vi "CAL_FLOW_SENSOR 2016.vi"(7 "Array in":refnum<k24>[](array[refnum]), 8 "error in (no error)":errorcluster, 9 "Descriptions":string[](array[string]), 11 "flow_slope_IN":dbl=51.35 format="%.2f") -> (0 "error out":errorcluster, 2 "Sensor Cluster":T1, 3 "flow_slope\nmL/min":dbl=51.35 format="%.2f", 5 "Array out":refnum<k24>[](array[refnum]))   [LabVIEW 2016]
uses:
  C:/Program Files (x86)/National Instruments/LabVIEW 2016/vi.lib/ULx/ULx_LV.dll
  Waterloo DAQ/controls/MCC DAQ Readings.ctl
  KPRO_lv2015/ad interface/Global_SIM_switch.vi
  KPRO_lv2015/Kpro Globals.vi
panel:
  out "Flow":dbl format="%.2f"
  in  "stop":bool
  in  "start":bool
  # "FLOW SENSOR CALIBRATION"
  # "Start Kpro flow. Allow the flow to equilibrate."
  # "After flow has equilibrated,  Press Start, simultaneously move Kpro effluent into graduated cylinder."
  # "Press Stop when 100 mL of water has been collected."
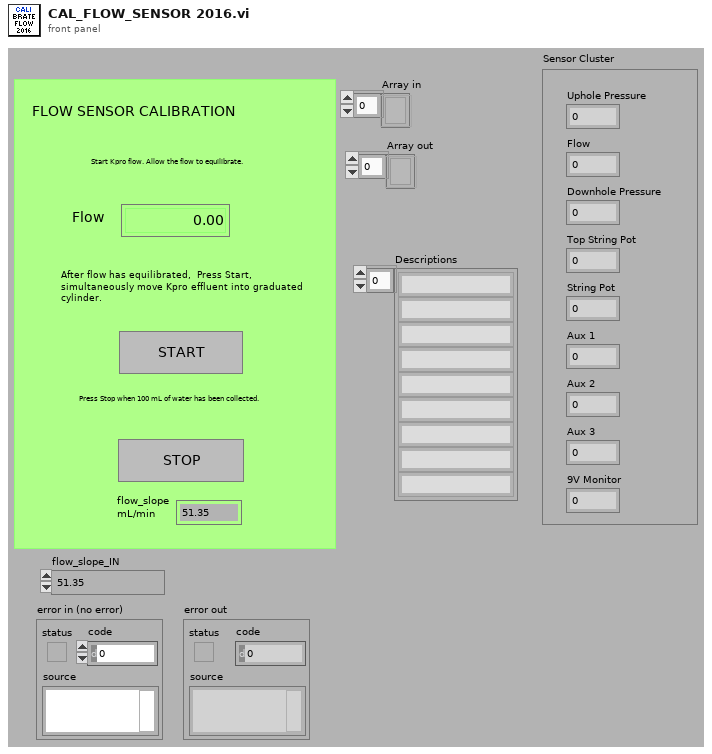
[diagram p1: front panel]
types:
  T1 = typedef "MCC DAQ Readings.ctl" = cluster{"Uphole Pressure":dbl, "Flow":dbl, "Downhole Pressure":dbl, "Top String Pot":dbl, "String Pot":dbl, "Aux 1":dbl, "Aux 2":dbl, "Aux 3":dbl, "9V Monitor":dbl}
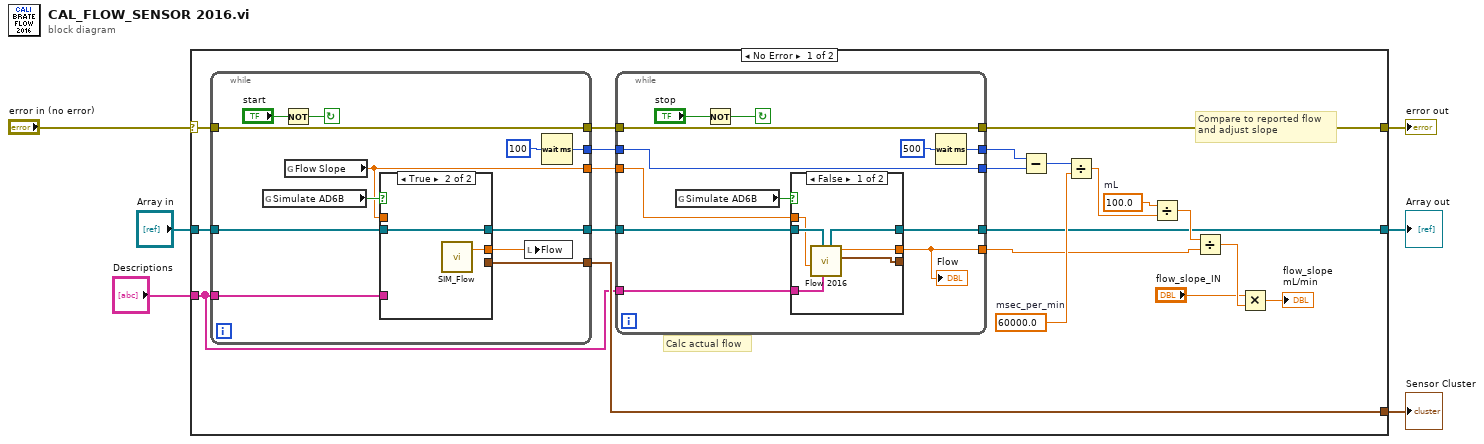
[diagram p0: block diagram]
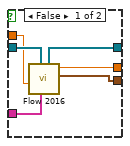
[diagram p2: hidden frame]
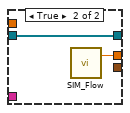
[diagram p3: hidden frame]
diagram:
  n1 = case shown="No Error" "error in (no error)" {
    selector: "error in (no error)" -> [w27 w69]
    tunnel: [w25 w69] -> w6
    tunnel: "Descriptions" -> [w10 _]
    tunnel: "Array in" -> [w12 w68]
    tunnel: [w11 _] -> w2
    tunnel: [w8 w68] -> w1
    frame No Error {
      w20 = 60000.0  # msec_per_min
      w21 = 100.0  # mL
      # "Compare to reported flow\nand adjust slope"
      # "Calc actual flow"
      n2 = while {
        tunnel: [w35] -> w26
        tunnel: w27 -> [w35]
        tunnel: [w36] -> w24
        tunnel: w10 -> [w32]
        tunnel: w12 -> [w31]
        tunnel: [w30] -> w11
        tunnel: [w29] -> w9
        tunnel: [w28] -> w7
        stop <- w38 continue-if-true
        n3 = global read "Global_SIM_switch.vi" "Simulate AD6B"() -> (w34:bool)
        n4 = Not(x="start") -> (.not. x?=w38:bool)
        n5 = global read "Kpro Globals.vi" "Flow Slope"() -> (w28:dbl)
        n6 = case shown="True" w34 {
          tunnel: [w42 w47] -> w33
          tunnel: w32 -> [w45 _]
          tunnel: w31 -> [w44 w46]
          tunnel: [w43 _] -> w30
          tunnel: w28 -> [w41 _]
          tunnel: [w40 w46] -> w29
          frame False {
            n7 = call "Flow 2016.vi"("Descriptions"=w45, "Array in"=w44, "Flow Slope"=w41) -> ("Sensor Cluster"=w43:T1, "Flow (ml/min)"=w42:dbl, "Array out"=w40:refnum<k24>[])  [unwired: 5 in]
          }
          frame True {
            n8 = call "SIM_Flow.vi"() -> ("Flow (ml/min)"=w47:dbl)  [unwired: 3 in]
          }
        }
        n9 = local write "Flow"(w33) -> ()
        n10 = Wait (ms)(milliseconds to wait=u32 100) -> (millisecond timer value=w36:u32)
      }
      n11 = while {
        tunnel: [w49] -> w13
        tunnel: w24 -> [w54]
        tunnel: [w54] -> w22
        tunnel: w26 -> [w55]
        tunnel: [w55] -> w25
        tunnel: [w57] -> w23
        tunnel: w10 -> [w52]
        tunnel: w9 -> [w51]
        tunnel: [w50] -> w8
        tunnel: w7 -> [w48]
        stop <- w59 continue-if-true
        n12 = global read "Global_SIM_switch.vi" "Simulate AD6B"() -> (w53:bool)
        n13 = Not(x="stop") -> (.not. x?=w59:bool)
        n14 = case shown="False" w53 {
          tunnel: [w62 w67] -> w49
          tunnel: w52 -> [w65 _]
          tunnel: w51 -> [w64 w66]
          tunnel: [w63 _] -> _
          tunnel: w48 -> [w61 _]
          tunnel: [w60 w66] -> w50
          frame False {
            n15 = call "Flow 2016.vi"("Descriptions"=w65, "Array in"=w64, "Flow Slope"=w61) -> ("Sensor Cluster"=w63:T1, "Flow (ml/min)"=w62:dbl, "Array out"=w60:refnum<k24>[])  [unwired: 5 in]
          }
          frame True {
            n16 = call "SIM_Flow.vi"() -> ("Flow (ml/min)"=w67:dbl)  [unwired: 3 in]
          }
        }
        "Flow" <- w49
        n17 = Wait (ms)(milliseconds to wait=u32 500) -> (millisecond timer value=w57:u32)
      }
      n18 = Subtract(x=w23, y=w22) -> (x-y=w19:u32)
      n19 = Divide(x=w19, y=w20) -> (x/y=w18:dbl)
      n20 = Divide(x=w21, y=w18) -> (x/y=w14:dbl)
      n21 = Divide(x=w14, y=w13) -> (x/y=w17:dbl)
      n22 = Multiply(x="flow_slope_IN", y=w17) -> (x*y=→"flow_slope\nmL/min":dbl)
    }
    frame Error {
    }
  }
  "error out" <- w6
  "Sensor Cluster" <- w2
  "Array out" <- w1
